vi "Set Trigger Mode.vi"(8 "error in (no error)":errorcluster, 10 "Trigger Mode":T1, 11 "MSOX6004 in":refnum<class "MSOX6004.lvclass">) -> (0 "error out":errorcluster, 3 "MSOX6004 out":refnum<class "MSOX6004.lvclass">)   [LabVIEW 2018, in "MSOX6004.lvlib" / "MSOX6004.lvclass"]
doc: "This Override sets the trigger to Auto or Normal mode. Auto generates a trigger even if one has not been detected after certain perios of time. Normal waits for trigger detection."
uses:
  MSOX6004.lvclass
  PPLs/Oscilloscope/Parent/Oscilloscope.lvlibp/Custom Controls/Trigger Mode.ctl
  MSOX6004.lvclass/MSOX6004.ctl
  <instrlib>/Keysight InfiniiVision/Keysight InfiniiVision.lvlib
  PPLs/Oscilloscope/Parent/Oscilloscope.lvlibp
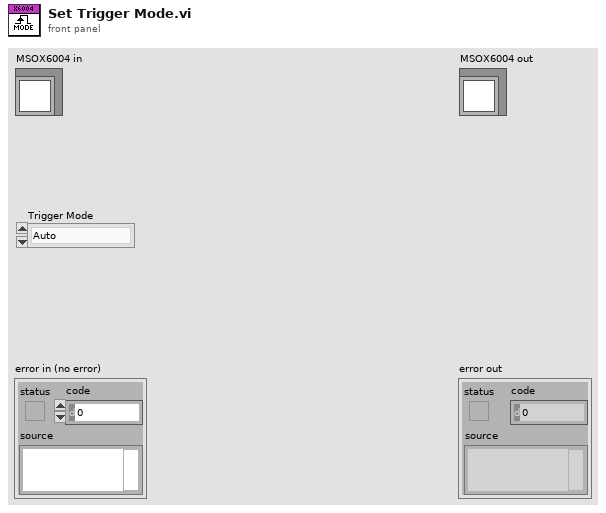
[diagram p1: front panel]
types:
  T1 = typedef "Oscilloscope.lvlibp/Trigger Mode.ctl" = enum16{"Auto", "Normal"}
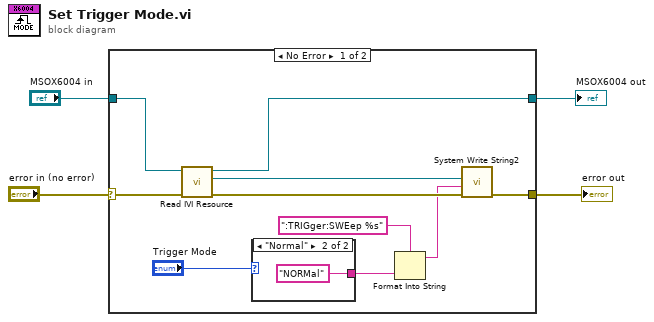
[diagram p0: block diagram]
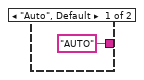
[diagram p2: hidden frame]
diagram:
  n1 = case shown="No Error" "error in (no error)" {
    selector: "error in (no error)" -> [w14 w18]
    tunnel: [w5 w18] -> w3
    tunnel: [w12 w17] -> w2
    tunnel: "MSOX6004 in" -> [w13 w17]
    frame No Error {
      n2 = call "Read IVI Resource.vi"("error in (no error)"=w14, "MSOX6004 in"=w13) -> ("error out"=w11:errorcluster, "IVI Resource"=w10:refnum<k15>, "MSOX6004 out"=w12:refnum<class "MSOX6004.lvclass">)  [unwired: 7 in]
      n3 = case shown="\"Normal\"" "Trigger Mode" {
        tunnel: ["AUTO" "NORMal"] -> w7
        frame "Auto", Default {
        }
        frame "Normal" {
        }
      }
      n4 = Format Into String(format string=":TRIGger:SWEep %s", w7) -> (resulting string=w6:string)  [unwired: 2 in, 1 out]
      n5 = call <instrlib>:"System Write String2.vi"("error in (no error)"=w11, "Data"=w6, "instrument handle"=w10) -> ("error out"=w5:errorcluster)  [unwired: 7 in, 1 out]
    }
    frame Error {
    }
  }
  "error out" <- w3
  "MSOX6004 out" <- w2
